vi "Stop.vi"(8 "error in (no error)":errorcluster, 11 "HAL GOOP4:Series Base in":refnum<class "Series Base.lvclass">) -> (0 "error out":errorcluster, 3 "HAL GOOP4:Series Base out":refnum<class "Series Base.lvclass">)   [LabVIEW 2023, in "HAL GOOP4.lvlib" / "Series Base.lvclass"]
uses:
  Series Base.lvclass
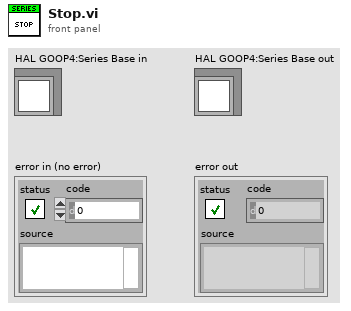
[diagram p1: front panel]
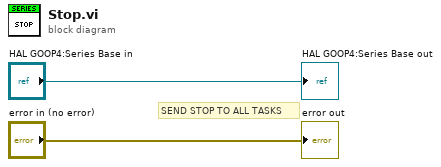
[diagram p0: block diagram]
diagram:
  # "SEND STOP TO ALL TASKS"
  "error out" <- "error in (no error)"
  "HAL GOOP4:Series Base out" <- "HAL GOOP4:Series Base in"
